vi "ESNsub_RLSupdate.vi"(7 "Settings":cluster{"lamda":dbl, "Delta":dbl}={"lamda"=0.995, "Delta"=0.001}, 8 "error in (no error)":errorcluster, 9 "e(n-1)":dbl[](array[numeric]), 10 "X(n)":dbl[](array[numeric]), 11 "W":T1) -> (0 "error out":errorcluster, 3 "Wn+1":T1)   [LabVIEW 2010]
uses:
  <vilib>/Analysis/Matrix/Datatypes/RealMatrix.ctl
  <vilib>/Analysis/Matrix/Numeric/Conversions/Array To Matrix - RA2.vi
  <vilib>/Analysis/baseanly.llb/A x Vector.vi
  <vilib>/Analysis/baseanly.llb/Real Dot Product.vi
  <vilib>/Analysis/baseanly.llb/Real Outer Product.vi
  <vilib>/Analysis/Matrix/Numeric/Add/Add - RM,RM.vi
  <vilib>/Analysis/baseanly.llb/Vector x A.vi
  <vilib>/Analysis/Matrix/Numeric/Subtract/Subtract - RM,RM.vi
  <vilib>/Analysis/Matrix/Numeric/Multiply/Multiply - RM,R.vi
  <vilib>/Analysis/NI_AALBase.lvlib
  <vilib>/Analysis/Matrix/NI_Matrix.lvlib
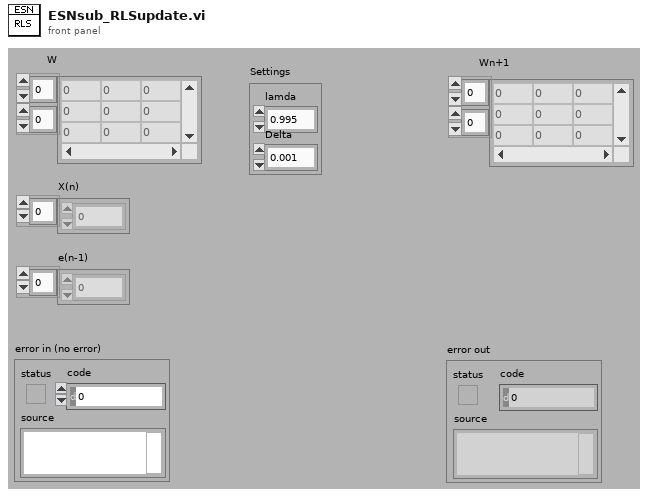
[diagram p1: front panel]
types:
  T1 = typedef "NI_Matrix.lvlib/RealMatrix.ctl" = dbl[][]
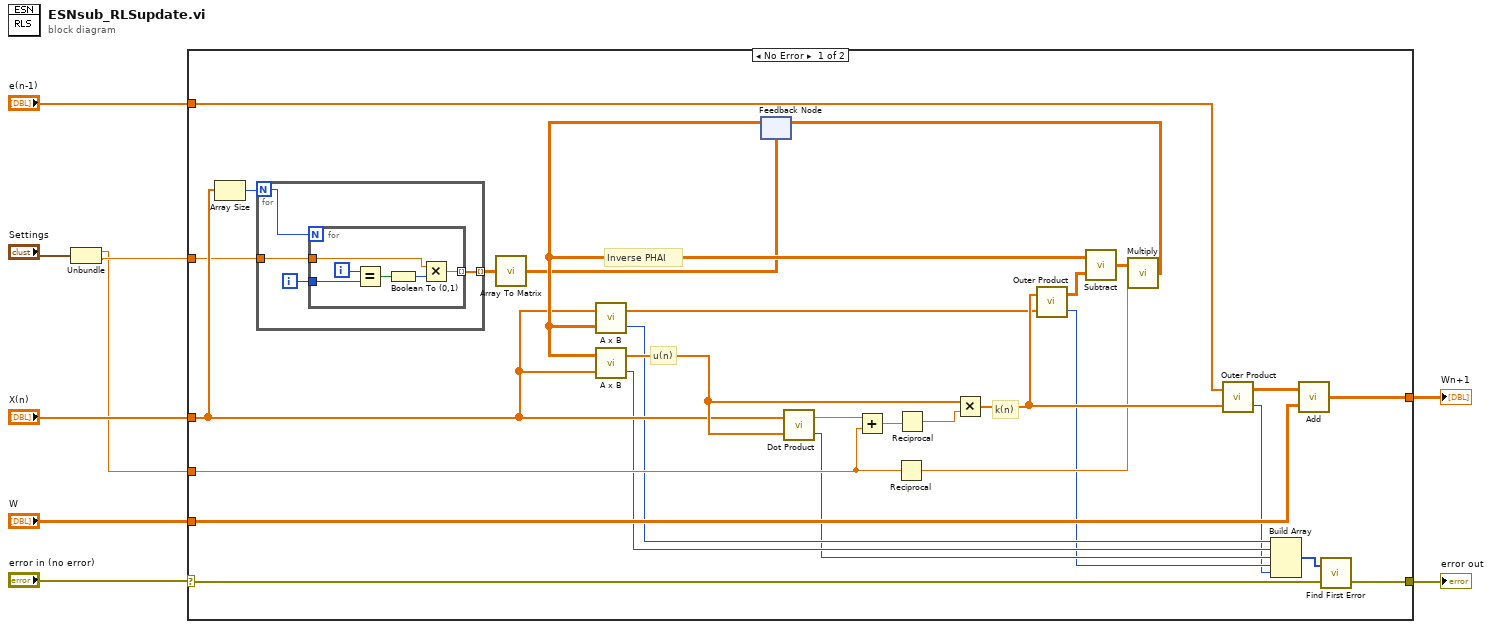
[diagram p0: block diagram]
diagram:
  n1 = Unbundle("Settings") -> ("lamda"=w3:dbl, "Delta"=w4:dbl)
  n2 = case shown="No Error" "error in (no error)" {
    selector: "error in (no error)" -> [w11 w50]
    tunnel: "e(n-1)" -> [w35 _]
    tunnel: [w33 w49] -> w8
    tunnel: "W" -> [w32 w49]
    tunnel: w3 -> [w28 _]
    tunnel: "X(n)" -> [w23 _]
    tunnel: w4 -> [w18 _]
    tunnel: [w10 w50] -> w1
    frame No Error {
      # "Inverse PHAI"
      # "k(n)"
      # "u(n)"
      n3 = Array Size(array=w23) -> (size(s)=w22:i32)
      n4 = for {
        N: w22 -> [w42]
        tunnel: w18 -> [w40]
        tunnel: [w39] -> w21 mode=indexing
        i -> [w41]
        n5 = for {
          N: w42 -> [_]
          tunnel: w41 -> [w47]
          tunnel: w40 -> [w44]
          tunnel: [w43] -> w39 mode=indexing
          i -> [w48]
          n6 = Equal?(x=w48, y=w47) -> (x = y?=w46:bool)
          n7 = Boolean To (0,1)(Boolean=w46) -> (0, 1=w45:i16)
          n8 = Multiply(x=w44, y=w45) -> (x*y=w43:dbl)
        }
      }
      n9 = call-poly <vilib>:"Array To Matrix.vi"("Real 2D Array"=w21) -> ("Real Matrix"=w19:T1)
      n10 = feedback #1(w19) -> (w25:T1)
      n11 = call-poly <vilib>:"A x B.vi"("Matrix A"=w25, "Vector V'"=w23) -> ("error"=w17:i32, "V' x A"=w30:dbl[])
      n12 = call-poly <vilib>:"A x B.vi"("Vector"=w23, "A"=w25) -> ("error"=w16:i32, "A x Vector"=w24:dbl[])
      n13 = call-poly <vilib>:"Dot Product.vi"("Y Vector"=w24, "X Vector"=w23) -> ("error"=w15:i32, "X * Y"=w38:dbl)
      n14 = Add ("Add.vi")(x=w38, y=w28) -> (x+y=w37:dbl)
      n15 = Reciprocal(x=w28) -> (1/x=w26:dbl)
      n16 = Reciprocal(x=w37) -> (1/x=w36:dbl)
      n17 = Multiply ("Multiply.vi")(x=w24, y=w36) -> (x*y=w31:dbl[])
      n18 = call-poly <vilib>:"Outer Product.vi"("Y Vector"=w30, "X Vector"=w31) -> ("error"=w14:i32, "Outer Product"=w29:T1)
      n19 = call-poly <vilib>:"Subtract.vi"("Real Matrix B"=w29, "Real Matrix A"=w25) -> ("A - B"=w27:T1)
      n20 = call-poly <vilib>:"Multiply.vi"("Real Scalar c"=w26, "Real Matrix A"=w27) -> ("A * c"=w20:T1)
      n21 = feedback-in #1(w20) -> ()
      n22 = call-poly <vilib>:"Outer Product.vi"("Y Vector"=w31, "X Vector"=w35) -> ("error"=w13:i32, "Outer Product"=w34:T1)
      n23 = Build Array(w17, w16, w15, w14, w13) -> (w12:i32[])
      n24 = call-poly <vilib>:"Add.vi"("Real Matrix B"=w32, "Real Matrix A"=w34) -> ("A + B"=w33:T1)
      n25 = call <vilib>:"Find First Error.vi"("error in (no error)"=w11, "error codes"=w12) -> ("error out"=w10:errorcluster)  [unwired: 2 in, 1 out]
    }
    frame Error {
    }
  }
  "Wn+1" <- w8
  "error out" <- w1
